vi "GetDistinctName.vi"(8 "error in (no error)":errorcluster, 10 "Proposed name":string="New Accessor 1", 11 "LVClassLibrary Refnum":refnum<vi>) -> (0 "error out":errorcluster, 2 "Accepted name":string, 3 "LVClassLibrary Refnum out":refnum<vi>)   [LabVIEW 2021, in "MemberVICreation.lvlib" / "BaseAccessorScripter.lvclass"]
uses:
  <resource>/Framework/Providers/LVClassLibrary/NewAccessors/BaseAccessorScripter/BaseAccessorScripter.lvclass
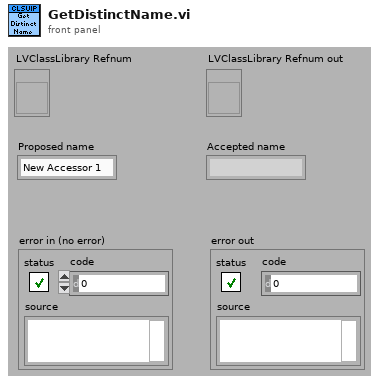
[diagram p1: front panel]
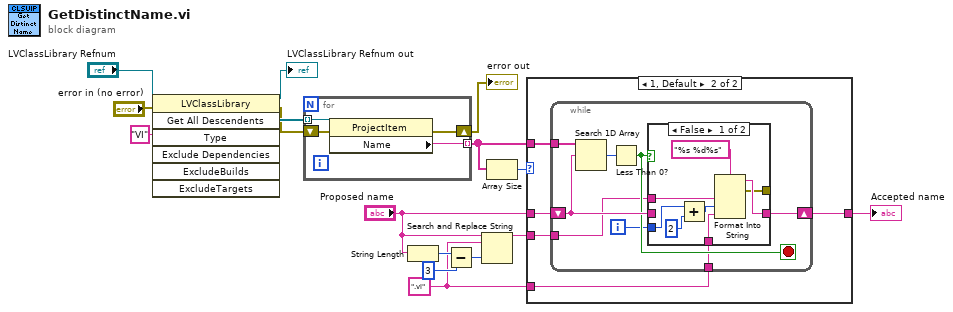
[diagram p0: block diagram]
diagram:
  w1 = ".vi" ("search string")
  n1 = invoke class="LVClassLibrary" method="Get All Descendents"(reference="LVClassLibrary Refnum", error in="error in (no error)", "Type"="VI") -> (reference out=→"LVClassLibrary Refnum out":refnum<vi>, error out=w11:errorcluster, "All Descendents"=w12:refnum<vi>[])  [unwired: 4 in, 4 out]
  n2 = for {
    tunnel: w12 -> [w20] mode=indexing
    shift-right: [w18] -> w9
    shift-left: w11 -> [w19]
    tunnel: [w17] -> w8 mode=indexing
    n3 = property class="ProjectItem"(reference=w20, error in=w19) -> (error out=w18:errorcluster, "Name"=w17:string)  [unwired: 1 out]
  }
  "error out" <- w9
  n4 = String Length(string="Proposed name") -> (length=w6:i32)
  n5 = Subtract(x=w6, y=3) -> (x-y=w5:i32)
  n6 = Search and Replace String(input string="Proposed name", search string=w1, offset=w5) -> (result string=w2:string)  [unwired: 1 in, 7 out]
  n7 = Array Size(array=w8) -> (size(s)=w7:i32)
  n8 = case shown="1, Default" w7 {
    tunnel: w8 -> [_ w26]
    tunnel: "Proposed name" -> [w21 w25]
    tunnel: [w21 w24] -> w10
    tunnel: w2 -> [_ w23]
    tunnel: w1 -> [_ w22]
    frame 0 {
    }
    frame 1, Default {
      n9 = while {
        tunnel: w26 -> [w34]
        shift-right: [w32] -> w24
        shift-left: w25 -> [w31]
        tunnel: w23 -> [w29]
        tunnel: w22 -> [w27]
        i -> [w28]
        stop <- w30 stop-if-true
        n10 = Search 1D Array(1D array=w34, element=w31) -> (index of element=w33:i32)  [unwired: 1 out]
        n11 = Less Than 0?(x=w33) -> (x < 0?=w30:bool)
        n12 = case shown="False" w30 {
          tunnel: [w40 w43] -> w32
          tunnel: w31 -> [_ w43]
          tunnel: w29 -> [w41 _]
          tunnel: w28 -> [w42 _]
          tunnel: [w39 _] -> _
          tunnel: w27 -> [w36 _]
          frame False {
            n13 = Add(x=w42, y=2) -> (x+y=w38:i32)
            n14 = Format Into String(format string="%s %d%s", w41, w38, w36) -> (resulting string=w40:string, error out=w39:errorcluster)  [unwired: 2 in]
          }
          frame True {
          }
        }
      }
    }
  }
  "Accepted name" <- w10
